vi "Parse Bitfile EST Clusters.vi"(8 "error in (no error)":errorcluster, 11 "bitfile path":path) -> (0 "error out":errorcluster, 1 "version":string, 2 "EPS IP LUT":variant, 3 "valid bitfile":bool, 4 "EST version enum":T1)   [LabVIEW 2020, in "Engine Simulation Toolkit System Explorer.lvlib"]
uses:
  Engine Simulation Toolkit System Explorer.lvlib
  Shared/Bitfile EST Version.ctl
  Shared/Properties.vi
  Shared/Engine Simulation Toolkit Shared.lvlib
  <vilib>/Utility/Data Type/NI_Data Type.lvlib
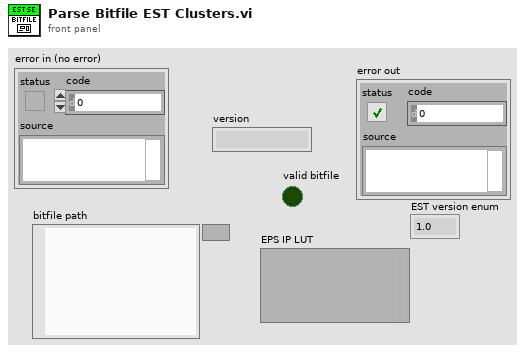
[diagram p1: front panel]
types:
  T1 = typedef "Engine Simulation Toolkit Shared.lvlib/Bitfile EST Version.ctl" = enum16{"1.0", "1.1", "1.2", "1.3", "1.4"}
  T2 = typedef "niFpgaBitfileStructure_VI.ctl" = cluster{"Name":string, "RegisterMap":T3[], "Icon":T8}
  T3 = typedef "nirviControlStructure.ctl" = cluster{"Name":string, "Hidden":bool, "Indicator":bool, "Flattened Type":string, "Grouping":cluster{"Grouped":bool, "Member Names":string[], "Member IDs":u32[]}, "Address":u32, "Size":u32, "Class":u32, "Internal":bool, "Typedef":T4, "ID":u32, "Bidirectional":bool, "Synchronous":bool, "Mechanical Action":T5, "Sub Controls":T6[], "Access May Timeout":bool, "Register Node":bool}
  T4 = typedef "nirviTypdefDescription.ctl" = cluster{"Typedef":bool, "Path":path}
  T5 = typedef "nirviMechanicalAction.ctl" = enum8{"Switch When Pressed", "Switch When Released", "Switch Until Released", "Latch When Pressed", "Latch When Released", "Latch Until Released"}
  T6 = typedef "nirviSubControlStructure.ctl" = cluster{"Name":string, "flattened Type":string, "Cluster Information":T7, "Typedef":T4}
  T7 = typedef "nirviClusterElementControl.ctl" = cluster{"Name Hierarchy":string[], "Item Order":u32[]}
  T8 = typedef "imagedata.ctl" = cluster{"image type":i32, "image depth":i32, "image":u8[], "mask":u8[], "colors":u32[], "Rectangle":cluster{"left":i16, "top":i16, "right":i16, "bottom":i16}}
  T9 = typedef "Engine Simulation Toolkit Shared.lvlib/IP Interface Enum.ctl" = enum16{"APU Settings", "APU Shared Settings", "APU Output", "APU Input", "Analog Replay Settings", "Analog Replay Load Input", "Analog Replay Input", "ETiming Capture Output", "ETiming Meas Settings", "ETiming Meas Output", "Digital PatGen Settings", "Digital PatGen Input", "Digital PatGen Load Input", "Knock Sensor Input", "Knock Sensor Settings", "Knock Cyl Input", "Knock Cyl Settings", "Dir Speed Input", "Dir Speed Settings", "Dir Speed Load Input", "APU Go"}
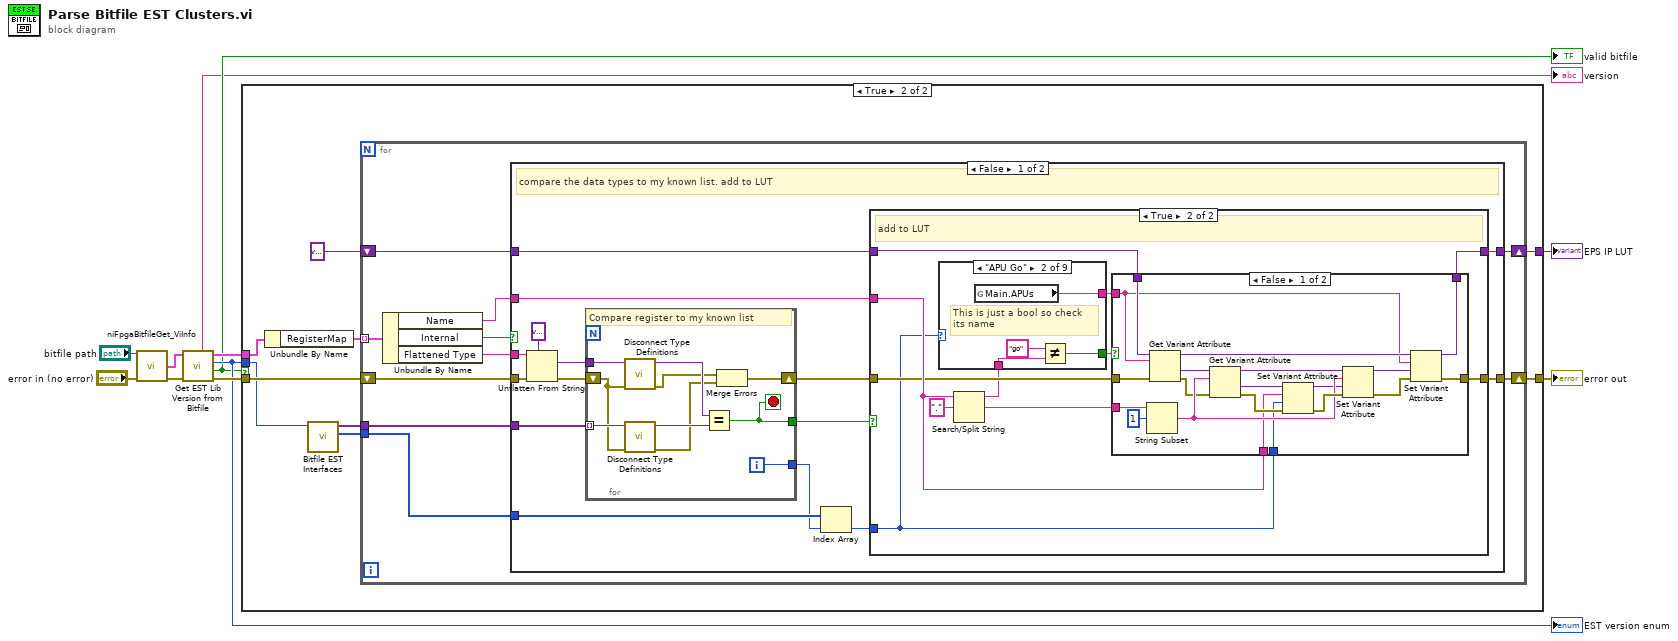
[diagram p0: block diagram]
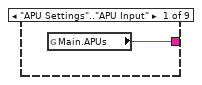
[diagram p5: hidden frame]
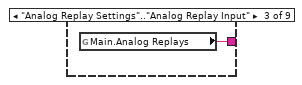
[diagram p6: hidden frame]
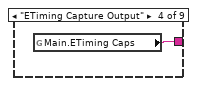
[diagram p7: hidden frame]
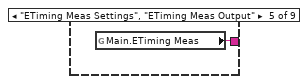
[diagram p8: hidden frame]
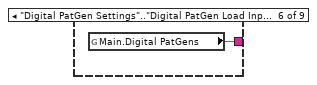
[diagram p9: hidden frame]
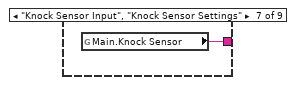
[diagram p10: hidden frame]
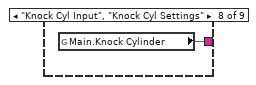
[diagram p11: hidden frame]
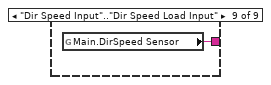
[diagram p12: hidden frame]
diagram:
  n1 = call <vilib>:"niFpgaBitfileGet_ViInfo.vi"("bitfile path"="bitfile path", "error in (no error)"="error in (no error)") -> ("vi info"=w5:T2, "error out"=w10:errorcluster)  [unwired: 1 in, 11 out]
  n2 = call "Get EST Lib Version from Bitfile.vi"("error in (no error)"=w10, "vi info"=w5) -> ("error out"=w6:errorcluster, "valid bitfile"=w2:bool, "EST version enum"=w3:T1, "vi info dup"=w4:T2, "EST version string"=→"version":string)  [unwired: 5 in]
  "valid bitfile" <- w2
  "EST version enum" <- w3
  n3 = case shown="True" w2 {
    tunnel: [w12 w18] -> w9
    tunnel: [_ w16] -> w7
    tunnel: w6 -> [w12 w15]
    tunnel: w4 -> [_ w14]
    tunnel: w3 -> [_ w13]
    frame False {
    }
    frame True {
      n4 = Unbundle By Name(w14) -> ("RegisterMap"=w21:T3[])
      n5 = call "Bitfile EST Interfaces.vi"("Version"=w13) -> ("IP Types"=w19:T9[], "IP Interface"=w20:variant[])  [unwired: 9 in]
      n6 = for {
        shift-right: [w31] -> w18
        shift-left: w15 -> [w28]
        tunnel: w21 -> [w30] mode=indexing
        tunnel: w20 -> [w25]
        tunnel: w19 -> [w24]
        shift-right: [w22] -> w16
        shift-left: variant ("Variant") -> [w23]
        n7 = Unbundle By Name(w30) -> ("Name"=w29:string, "Internal"=w26:bool, "Flattened Type"=w27:string)
        n8 = case shown="False" w26 {
          tunnel: [w37 w105] -> w31
          tunnel: w29 -> [w36 _]
          tunnel: w28 -> [w45 w105]
          tunnel: w27 -> [w43 _]
          tunnel: w25 -> [w41 _]
          tunnel: w24 -> [w40 _]
          tunnel: w23 -> [w39 w104]
          tunnel: [w38 w104] -> w22
          frame False {
            # "compare the data types to my known list. add to LUT"
            n9 = Unflatten From String(type=variant ("Variant"), binary string=w43, error in (no error)=w45) -> (value=w42:variant, error out=w46:errorcluster)  [unwired: 3 out]
            n10 = for {
              shift-right: [w96] -> w32
              shift-left: w46 -> [w97]
              tunnel: w42 -> [w99]
              tunnel: w41 -> [w98] mode=indexing
              tunnel: [w100] -> w33
              tunnel: [w103] -> w35
              i -> [w103]
              stop <- w100 stop-if-true
              # "Compare register to my known list"
              n11 = call <vilib>:"Disconnect Type Definitions.vi"("error in (no error)"=w97, "variant in"=w99) -> ("error out"=w95:errorcluster, "variant out"=w102:variant)  [unwired: 8 in]
              n12 = call <vilib>:"Disconnect Type Definitions.vi"("error in (no error)"=w97, "variant in"=w98) -> ("error out"=w94:errorcluster, "variant out"=w101:variant)  [unwired: 8 in]
              n13 = Equal?(x=w102, y=w101) -> (x = y?=w100:bool)
              n14 = Merge Errors(w95, w94) -> (w96:errorcluster)
            }
            n15 = Index Array(array=w40, index=w35) -> (element=w34:T9)
            n16 = case shown="True" w33 {
              tunnel: w34 -> [_ w51]
              tunnel: w39 -> [w47 w55]
              tunnel: [w47 w53] -> w38
              tunnel: w36 -> [_ w57]
              tunnel: [w48 w54] -> w37
              tunnel: w32 -> [w48 w56]
              frame False {
              }
              frame True {
                # "add to LUT"
                n17 = Search/Split String(string=w57, search string/char (-)=".") -> (substring before match=w50:string, match + rest of string=w58:string)  [unwired: 1 in, 1 out]
                n18 = case shown="\"APU Go\"" w51 {
                  tunnel: [w82 w86 w87 w88 w89 w90 w91 w92 w93] -> w52
                  tunnel: w50 -> [_ w85 _ _ _ _ _ _ _]
                  tunnel: [_ w83 _ _ _ _ _ _ _] -> w49
                  frame "APU Settings".."APU Input" {
                    n19 = global read "Properties.vi" "Main.APUs"() -> (w82:string)
                  }
                  frame "APU Go" {
                    # "This is just a bool so check its name"
                    n20 = global read "Properties.vi" "Main.APUs"() -> (w86:string)
                    n21 = Not Equal?(x="go", y=w85) -> (x != y?=w83:bool)
                  }
                  frame "Analog Replay Settings".."Analog Replay Input" {
                    n22 = global read "Properties.vi" "Main.Analog Replays"() -> (w87:string)
                  }
                  frame "ETiming Capture Output" {
                    n23 = global read "Properties.vi" "Main.ETiming Caps"() -> (w88:string)
                  }
                  frame "ETiming Meas Settings", "ETiming Meas Output" {
                    n24 = global read "Properties.vi" "Main.ETiming Meas"() -> (w89:string)
                  }
                  frame "Digital PatGen Settings".."Digital PatGen Load Input" {
                    n25 = global read "Properties.vi" "Main.Digital PatGens"() -> (w90:string)
                  }
                  frame "Knock Sensor Input", "Knock Sensor Settings" {
                    n26 = global read "Properties.vi" "Main.Knock Sensor"() -> (w91:string)
                  }
                  frame "Knock Cyl Input", "Knock Cyl Settings" {
                    n27 = global read "Properties.vi" "Main.Knock Cylinder"() -> (w92:string)
                  }
                  frame "Dir Speed Input".."Dir Speed Load Input" {
                    n28 = global read "Properties.vi" "Main.DirSpeed Sensor"() -> (w93:string)
                  }
                }
                n29 = case shown="False" w49 {
                  tunnel: w58 -> [w79 _]
                  tunnel: w57 -> [w71 _]
                  tunnel: w56 -> [w69 w81]
                  tunnel: w55 -> [w66 w80]
                  tunnel: [w65 w81] -> w54
                  tunnel: [w63 w80] -> w53
                  tunnel: w52 -> [w61 _]
                  tunnel: w51 -> [w60 _]
                  frame False {
                    n30 = String Subset(string=w79, offset (0)=1) -> (substring=w74:string)  [unwired: 1 in]
                    n31 = Get Variant Attribute(Variant=w66, name=w61, error in=w69) -> (duplicate Variant=w64:variant, value=w67:variant, error out=w68:errorcluster)  [unwired: 1 in, 1 out]
                    n32 = Get Variant Attribute(Variant=w67, name=w74, error in=w68) -> (duplicate Variant=w72:variant, value=w76:variant, error out=w77:errorcluster)  [unwired: 1 in, 1 out]
                    n33 = Set Variant Attribute(Variant=w76, name=w71, value=w60, error in=w77) -> (Variant out=w73:variant, error out=w75:errorcluster)  [unwired: 1 out]
                    n34 = Set Variant Attribute(Variant=w72, name=w74, value=w73, error in=w75) -> (Variant out=w62:variant, error out=w70:errorcluster)  [unwired: 1 out]
                    n35 = Set Variant Attribute(Variant=w64, name=w61, value=w62, error in=w70) -> (Variant out=w63:variant, error out=w65:errorcluster)  [unwired: 1 out]
                  }
                  frame True {
                  }
                }
              }
            }
          }
          frame True {
            # "avoid internal registers. They don't have a type and users didnt make them anyway"
          }
        }
      }
    }
  }
  "error out" <- w9
  "EPS IP LUT" <- w7
